vi "Float2Words.vi"(4 "value":sgl) -> (1 "output":u16[](array[numeric]))   [LabVIEW 2020, in "SMCD14_lib.lvlib"]
uses:
  SMCD14_lib.lvlib
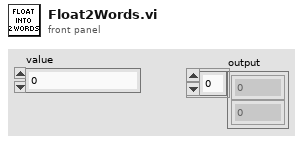
[diagram p1: front panel]
types:
  T1 = enum16{"big-endian, network order", "native, host order", "little-endian"}
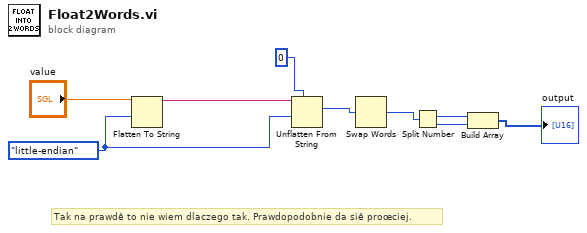
[diagram p0: block diagram]
diagram:
  w8 = T1."little-endian" ("byte order (0:big-endian, network order)")
  # "Tak na prawdê to nie wiem dlaczego tak. Prawdopodobnie da siê proœciej."
  n1 = Flatten To String(anything="value", byte order (0:big-endian, network order)=w8) -> (data string=w7:string)  [unwired: 2 in, 2 out]
  n2 = Unflatten From String(type=u32 0, binary string=w7, byte order (0:big-endian, network order)=w8) -> (value=w5:u32)  [unwired: 2 in, 2 out]
  n3 = Swap Words(1:w5) -> (0:w4:u32)
  n4 = Split Number(x=w4) -> (hi(x)=w3:u16, lo(x)=w2:u16)
  n5 = Build Array(w3, w2) -> (→"output":u16[])
